vi "TDS DCPS Set Output State.vi"(8 "error in (no error)":errorcluster, 9 "Output State":bool, 10 "Signal InstConfig":string, 11 "Address":string) -> (0 "error out":errorcluster)   [LabVIEW 2025, in "Interface Functions.lvlib"]
uses:
  Interface Functions.lvlib
panel:
  # "DCPS Set Output State"
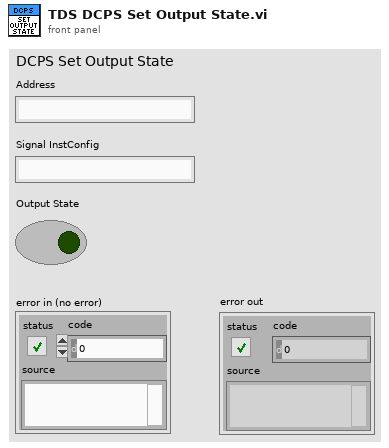
[diagram p1: front panel]
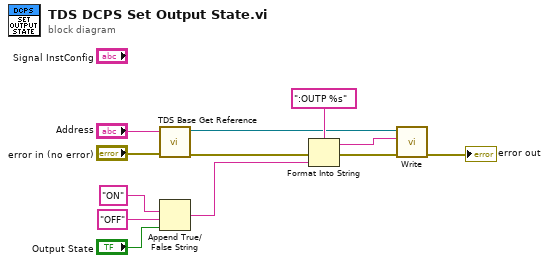
[diagram p0: block diagram]
diagram:
  n1 = call "TDS Base Get Reference.vi"("error in (no error)"="error in (no error)", "Address"="Address") -> ("error out"=w3:errorcluster, "Reference"=w4:refnum<visa-resource-name>)  [unwired: 8 in]
  n2 = Append True/False String(1:"Output State", 2:"OFF", 3:"ON") -> (0:w10:string)  [unwired: 1 out]
  n3 = Format Into String(format string=":OUTP %s", error in=w3, w10) -> (resulting string=w6:string, error out=w5:errorcluster)  [unwired: 1 in]
  n4 = call "Write.vi"("error in (no error)"=w5, "Write Buffer (\"\")"=w6, "VISA resource name"=w4) -> ("error out"=→"error out":errorcluster)  [unwired: 7 in, 1 out]
